vi "Folder& File Path.vi"(9 "File Name":string="Config.bin", 10 "Folder Name":string="Product config") -> (3 "appended path":path)   [LabVIEW 2015]
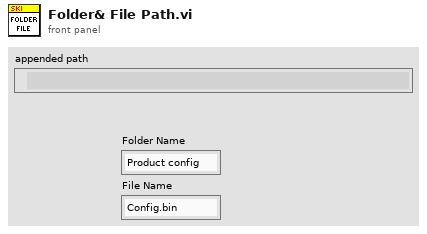
[diagram p1: front panel]
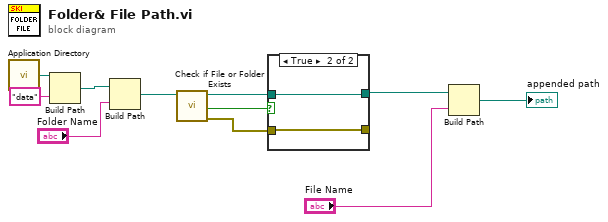
[diagram p0: block diagram]
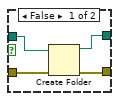
[diagram p2: hidden frame]
diagram:
  n1 = call <vilib>:"Application Directory.vi"() -> ("Application Directory"=w1:path)
  n2 = Build Path(base path=w1, name or relative path="data") -> (appended path=w3:path)
  n3 = Build Path(base path=w3, name or relative path="Folder Name") -> (appended path=w5:path)
  n4 = call <vilib>:"Check if File or Folder Exists.vi"("path"=w5) -> ("error out"=w8:errorcluster, "file or folder exists?"=w6:bool, "dup path"=w7:path)  [unwired: 8 in]
  n5 = case shown="True" w6 {
    tunnel: w7 -> [w15 w17]
    tunnel: w8 -> [w14 w16]
    tunnel: [w13 w17] -> w9
    tunnel: [w12 w16] -> _
    frame False {
      n6 = Create Folder(path (use dialog)=w15, error in=w14) -> (created path=w13:path, error out=w12:errorcluster)  [unwired: 1 in, 1 out]
    }
    frame True {
    }
  }
  n7 = Build Path(base path=w9, name or relative path="File Name") -> (appended path=→"appended path":path)
